vi "settings handler.vi"(7 "Operation":enum16{"Open", "Write", "Read", "Close"}(ring), 8 "error in (no error)":errorcluster, 9 "Paths write":cluster{"Android":path, "Version":path}, 11 "Write":T1={"COM"="", "baud rate"=115200, "data bits"=8, "parity"=enum."None", "stop bits"=10, "flow control"=enum."None", "delay"=50, "I/O channel"=""} {"stop bits" items=["1.0"=10, "1.5"=15, "2.0"=20]; "baud rate" max=921600; "data bits" max=16}) -> (0 "Error Out":errorcluster, 1 "Paths read":cluster{"Android":path, "Version":path}, 3 "Read":T1={"COM"="", "baud rate"=115200, "data bits"=8, "parity"=enum."None", "stop bits"=10, "flow control"=enum."None", "delay"=50, "I/O channel"=""} {"stop bits" items=["1.0"=10, "1.5"=15, "2.0"=20]; "baud rate" max=921600; "data bits" max=16})   [LabVIEW 2021]
uses:
  <vilib>/Utility/config.llb/Write Key (String).vi
  <vilib>/Utility/config.llb/Read Key (String).vi
  <vilib>/Utility/config.llb/Read Key (U32).vi
  <vilib>/Utility/config.llb/NI_LVConfig.lvlib
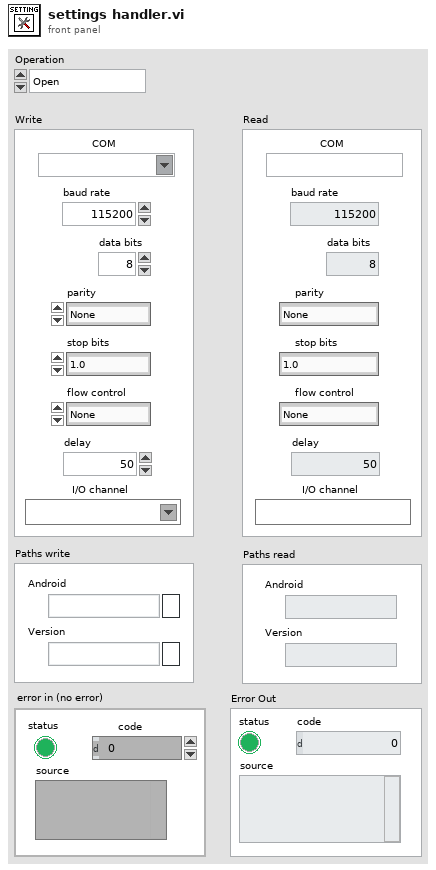
[diagram p1: front panel]
types:
  T1 = cluster{"COM":refnum<visa-resource-name>, "baud rate":u32, "data bits":u8, "parity":enum16{"None", "Odd", "Even", "Mark", "Space"}, "stop bits":u16, "flow control":enum16{"None", "XON/XOFF", "RTS/CTS", "DTR/DSR"}, "delay":u16, "I/O channel":refnum<k21>}
  T2 = typedef "NI_LVConfig.lvlib/Config Data RefNum.ctl" = refnum<k1>
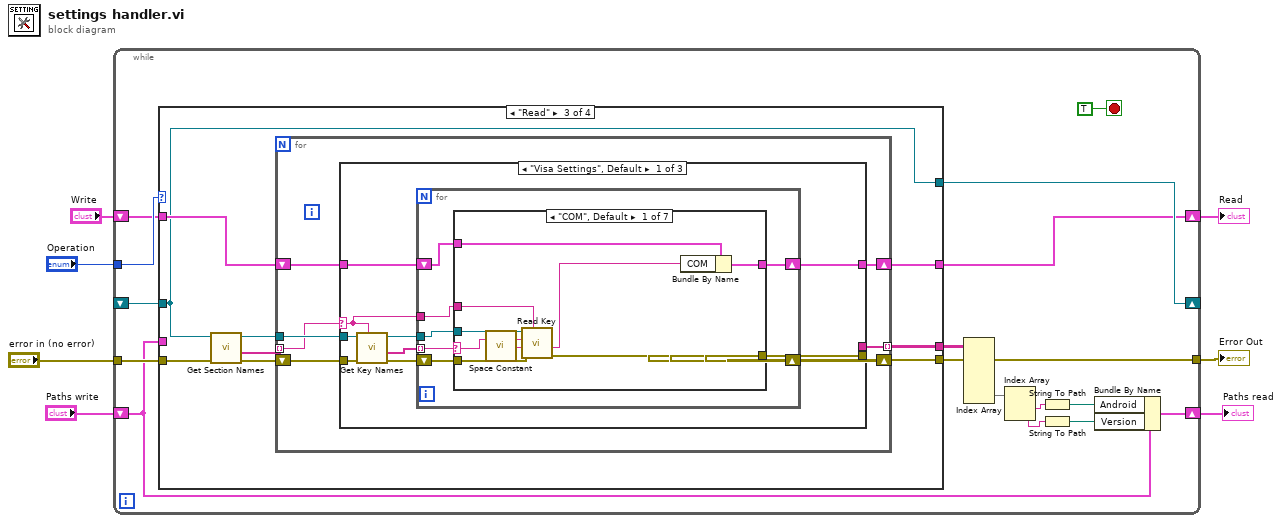
[diagram p0: block diagram]
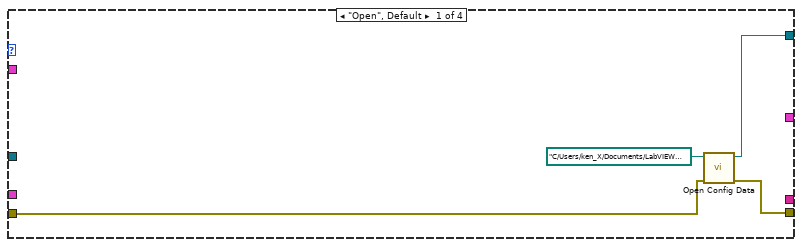
[diagram p2: hidden frame]
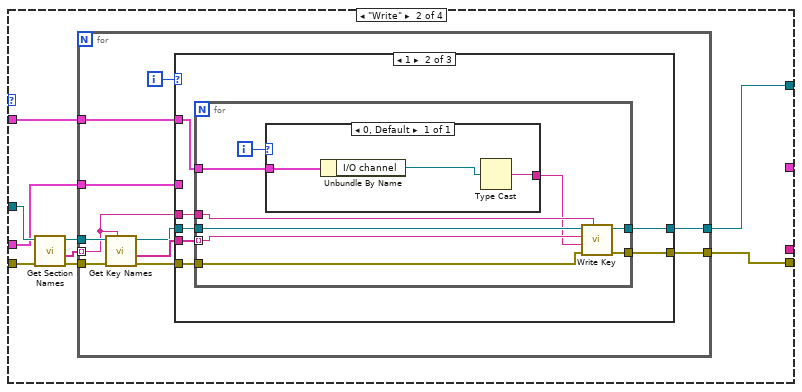
[diagram p3: hidden frame]
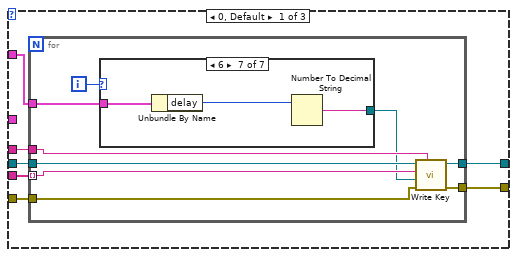
[diagram p4: hidden frame]
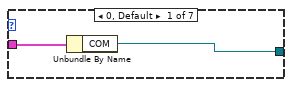
[diagram p5: hidden frame]
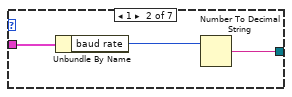
[diagram p6: hidden frame]
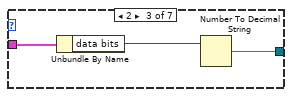
[diagram p7: hidden frame]
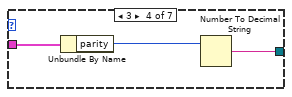
[diagram p8: hidden frame]
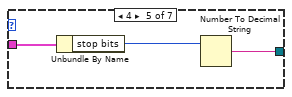
[diagram p9: hidden frame]
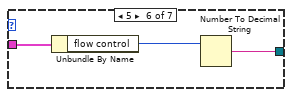
[diagram p10: hidden frame]
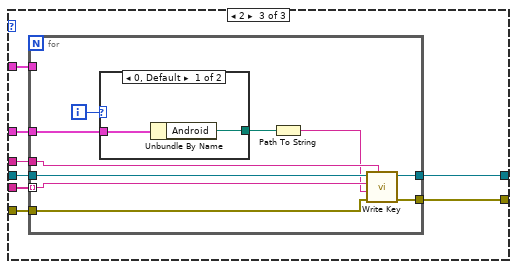
[diagram p11: hidden frame]
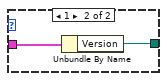
[diagram p12: hidden frame]
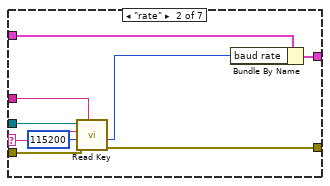
[diagram p13: hidden frame]
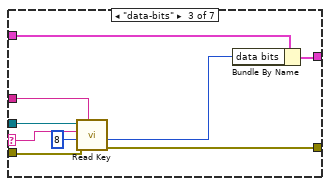
[diagram p14: hidden frame]
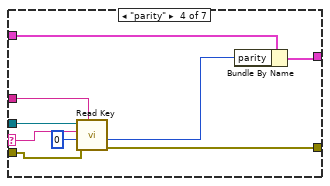
[diagram p15: hidden frame]
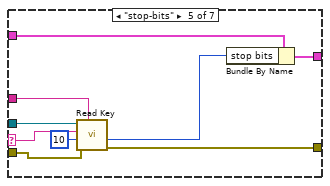
[diagram p16: hidden frame]
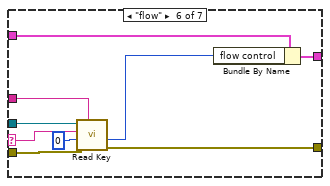
[diagram p17: hidden frame]
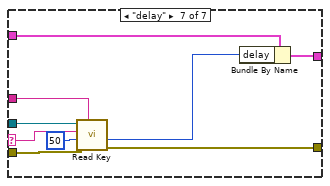
[diagram p18: hidden frame]
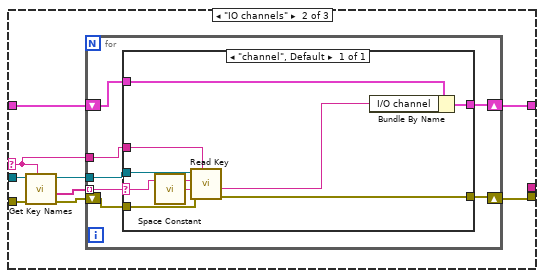
[diagram p19: hidden frame]
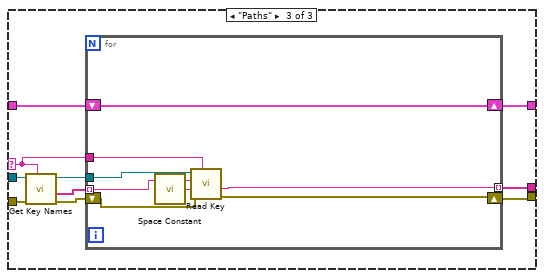
[diagram p20: hidden frame]
diagram:
  n1 = while {
    tunnel: "error in (no error)" -> [w23]
    tunnel: [w22] -> w6
    shift-right: [w21] -> _
    shift-left: _ -> [w19]
    shift-right: [w12] -> w3
    shift-left: "Write" -> [w17]
    tunnel: "Operation" -> [w18]
    shift-right: [w15] -> w1
    shift-left: "Paths write" -> [w16]
    stop <- TRUE stop-if-true
    n2 = case shown="\"Read\"" w18 {
      tunnel: w23 -> [w26 w33 w133 w265]
      tunnel: [w25 w29 w130 w264] -> w22
      tunnel: [w24 w30 w125 _] -> w21
      tunnel: w19 -> [_ w32 w125 w263]
      tunnel: w17 -> [_ w31 w128 _]
      tunnel: w16 -> [_ w28 _ _]
      tunnel: [_ _ w129 _] -> w12
      tunnel: [_ _ w127 _] -> w11
      frame "Open", Default {
        n3 = call <vilib>:"Open Config Data.vi"("error in (no error)"=w26, "configuration file path"=path "C:/Users/ken_X/Documents/LabVIEW projects/Project-A/settings/settings.ini" ("file path (use dialog)")) -> ("error out"=w25:errorcluster, "refnum"=w24:T2)  [unwired: 7 in, 1 out]
      }
      frame "Write" {
        n4 = call <vilib>:"Get Section Names.vi"("error in (no error)"=w33, "refnum"=w32) -> ("error out"=w34:errorcluster, "section names"=w36:string[], "refnum out"=w35:T2)  [unwired: 7 in]
        n5 = for {
          tunnel: w36 -> [w45] mode=indexing
          tunnel: w35 -> [w47]
          tunnel: w34 -> [w46]
          tunnel: [w41] -> w30
          tunnel: [w40] -> w29
          tunnel: w31 -> [w39]
          tunnel: w28 -> [w37]
          i -> [w38]
          n6 = call <vilib>:"Get Key Names.vi"("section"=w45, "error in (no error)"=w46, "refnum"=w47) -> ("error out"=w42:errorcluster, "key names"=w44:string[], "refnum out"=w43:T2)  [unwired: 5 in, 1 out]
          n7 = case shown="1" w38 {
            tunnel: w45 -> [w54 w90 w110]
            tunnel: w44 -> [w53 w89 w109]
            tunnel: w43 -> [w52 w88 w108]
            tunnel: w42 -> [w51 w87 w107]
            tunnel: [w50 w86 w106] -> w41
            tunnel: [w49 w85 w105] -> w40
            tunnel: w39 -> [w48 w84 w104]
            tunnel: w37 -> [_ _ w103]
            frame 0, Default {
              n8 = for {
                tunnel: w54 -> [w63]
                tunnel: w53 -> [w62] mode=indexing
                tunnel: w52 -> [w61]
                tunnel: w51 -> [w60]
                tunnel: [w59] -> w50
                tunnel: [w58] -> w49
                tunnel: w48 -> [w56]
                i -> [w57]
                n9 = case shown="6" w57 {
                  tunnel: w56 -> [w65 w68 w71 w74 w77 w80 w83]
                  tunnel: [w64 w66 w69 w72 w75 w78 w81] -> w55
                  frame 0, Default {
                    n10 = Unbundle By Name(w65) -> ("COM"=w64:refnum<visa-resource-name>)
                  }
                  frame 1 {
                    n11 = Unbundle By Name(w68) -> ("baud rate"=w67:u32)
                    n12 = Number To Decimal String(number=w67) -> (decimal integer string=w66:string)  [unwired: 1 in]
                  }
                  frame 2 {
                    n13 = Unbundle By Name(w71) -> ("data bits"=w70:u8)
                    n14 = Number To Decimal String(number=w70) -> (decimal integer string=w69:string)  [unwired: 1 in]
                  }
                  frame 3 {
                    n15 = Unbundle By Name(w74) -> ("parity"=w73:enum16{"None", "Odd", "Even", "Mark", "Space"})
                    n16 = Number To Decimal String(number=w73) -> (decimal integer string=w72:string)  [unwired: 1 in]
                  }
                  frame 4 {
                    n17 = Unbundle By Name(w77) -> ("stop bits"=w76:u16)
                    n18 = Number To Decimal String(number=w76) -> (decimal integer string=w75:string)  [unwired: 1 in]
                  }
                  frame 5 {
                    n19 = Unbundle By Name(w80) -> ("flow control"=w79:enum16{"None", "XON/XOFF", "RTS/CTS", "DTR/DSR"})
                    n20 = Number To Decimal String(number=w79) -> (decimal integer string=w78:string)  [unwired: 1 in]
                  }
                  frame 6 {
                    n21 = Unbundle By Name(w83) -> ("delay"=w82:u16)
                    n22 = Number To Decimal String(number=w82) -> (decimal integer string=w81:string)  [unwired: 1 in]
                  }
                }
                n23 = call-poly <vilib>:"Write Key.vi"("section"=w63, "error in (no error)"=w60, "value"=w55, "key"=w62, "refnum"=w61) -> ("error out"=w58:errorcluster, "refnum out"=w59:T2)  [unwired: 4 in, 1 out]
              }
            }
            frame 1 {
              n24 = for {
                tunnel: w90 -> [w99]
                tunnel: w89 -> [w98] mode=indexing
                tunnel: w88 -> [w97]
                tunnel: w87 -> [w96]
                tunnel: [w95] -> w86
                tunnel: [w94] -> w85
                tunnel: w84 -> [w92]
                i -> [w93]
                n25 = case shown="0, Default" w93 {
                  tunnel: w92 -> [w102]
                  tunnel: [w101] -> w91
                  frame 0, Default {
                    n26 = Unbundle By Name(w102) -> ("I/O channel"=w100:refnum<k21>)
                    n27 = Type Cast(x=w100) -> (*(type *) &x=w101:string)  [unwired: 1 in]
                  }
                }
                n28 = call-poly <vilib>:"Write Key.vi"("section"=w99, "error in (no error)"=w96, "value"=w91, "key"=w98, "refnum"=w97) -> ("error out"=w94:errorcluster, "refnum out"=w95:T2)  [unwired: 4 in, 1 out]
              }
            }
            frame 2 {
              n29 = for {
                tunnel: w110 -> [w120]
                tunnel: w109 -> [w119] mode=indexing
                tunnel: w108 -> [w118]
                tunnel: w107 -> [w117]
                tunnel: [w116] -> w106
                tunnel: [w115] -> w105
                tunnel: w104 -> [_]
                tunnel: w103 -> [w113]
                i -> [w114]
                n30 = case shown="0, Default" w114 {
                  tunnel: w113 -> [w121 w124]
                  tunnel: [w122 w123] -> w112
                  frame 0, Default {
                    n31 = Unbundle By Name(w121) -> ("Android"=w122:path)
                  }
                  frame 1 {
                    n32 = Unbundle By Name(w124) -> ("Version"=w123:path)
                  }
                }
                n33 = Path To String(path=w112) -> (string=w111:string)
                n34 = call-poly <vilib>:"Write Key.vi"("section"=w120, "error in (no error)"=w117, "value"=w111, "key"=w119, "refnum"=w118) -> ("error out"=w115:errorcluster, "refnum out"=w116:T2)  [unwired: 4 in, 1 out]
              }
            }
          }
        }
      }
      frame "Read" {
        n35 = call <vilib>:"Get Section Names.vi"("error in (no error)"=w133, "refnum"=w125) -> ("error out"=w131:errorcluster, "section names"=w132:string[], "refnum out"=w126:T2)  [unwired: 7 in]
        n36 = for {
          tunnel: w132 -> [w138] mode=indexing
          tunnel: w126 -> [w140]
          shift-right: [w137] -> w130
          shift-left: w131 -> [w139]
          shift-right: [w136] -> w129
          shift-left: w128 -> [w135]
          tunnel: [w134] -> w127 mode=indexing
          n37 = case shown="\"Visa Settings\", Default" w138 {
            selector: w138 -> [w144 w223 w249]
            tunnel: w140 -> [w149 w228 w254]
            tunnel: w139 -> [w148 w227 w253]
            tunnel: [w143 w222 w248] -> w137
            tunnel: [w142 w220 w246] -> w136
            tunnel: w135 -> [w141 w221 w247]
            tunnel: [_ _ w245] -> w134
            frame "Visa Settings", Default {
              n38 = call <vilib>:"Get Key Names.vi"("section"=w144, "error in (no error)"=w148, "refnum"=w149) -> ("error out"=w145:errorcluster, "key names"=w147:string[], "refnum out"=w146:T2)  [unwired: 5 in, 1 out]
              n39 = for {
                tunnel: w144 -> [w155]
                tunnel: w147 -> [w156] mode=indexing
                tunnel: w146 -> [w154]
                shift-right: [w152] -> w143
                shift-left: w145 -> [w153]
                shift-right: [w151] -> w142
                shift-left: w141 -> [w150]
                n40 = case shown="\"COM\", Default" w156 {
                  selector: w156 -> [w164 w173 w182 w191 w200 w209 w218]
                  tunnel: w155 -> [w165 w174 w183 w192 w201 w210 w219]
                  tunnel: w154 -> [w163 w172 w181 w184 w199 w208 w217]
                  tunnel: w153 -> [w162 w171 w180 w189 w197 w207 w216]
                  tunnel: [w160 w169 w178 w188 w196 w205 w214] -> w152
                  tunnel: w150 -> [w158 w168 w176 w186 w194 w203 w212]
                  tunnel: [w159 w167 w177 w187 w195 w204 w213] -> w151
                  frame "COM", Default {
                    n41 = call <vilib>:"Space Constant.vi"() -> ("String"=w161:string)
                    n42 = call-poly <vilib>:"Read Key.vi"("section"=w165, "error in (no error)"=w162, "default value"=w161, "key"=w164, "refnum"=w163) -> ("error out"=w160:errorcluster, "value"=w157:string)  [unwired: 3 in, 2 out]
                    n43 = Bundle By Name(cluster=w158, "COM"=w157) -> (w159:T1)
                  }
                  frame "rate" {
                    n44 = call-poly <vilib>:"Read Key.vi"("section"=w174, "error in (no error)"=w171, "default value"=u32 115200, "key"=w173, "refnum"=w172) -> ("error out"=w169:errorcluster, "value"=w166:u32)  [unwired: 3 in, 2 out]
                    n45 = Bundle By Name(cluster=w168, "baud rate"=w166) -> (w167:T1)
                  }
                  frame "data-bits" {
                    n46 = call-poly <vilib>:"Read Key.vi"("section"=w183, "error in (no error)"=w180, "default value"=u32 8, "key"=w182, "refnum"=w181) -> ("error out"=w178:errorcluster, "value"=w175:u32)  [unwired: 3 in, 2 out]
                    n47 = Bundle By Name(cluster=w176, "data bits"=w175) -> (w177:T1)
                  }
                  frame "parity" {
                    n48 = call-poly <vilib>:"Read Key.vi"("section"=w192, "error in (no error)"=w189, "default value"=u32 0, "key"=w191, "refnum"=w184) -> ("error out"=w188:errorcluster, "value"=w185:u32)  [unwired: 3 in, 2 out]
                    n49 = Bundle By Name(cluster=w186, "parity"=w185) -> (w187:T1)
                  }
                  frame "stop-bits" {
                    n50 = call-poly <vilib>:"Read Key.vi"("section"=w201, "error in (no error)"=w197, "default value"=u32 10, "key"=w200, "refnum"=w199) -> ("error out"=w196:errorcluster, "value"=w193:u32)  [unwired: 3 in, 2 out]
                    n51 = Bundle By Name(cluster=w194, "stop bits"=w193) -> (w195:T1)
                  }
                  frame "flow" {
                    n52 = call-poly <vilib>:"Read Key.vi"("section"=w210, "error in (no error)"=w207, "default value"=u32 0, "key"=w209, "refnum"=w208) -> ("error out"=w205:errorcluster, "value"=w202:u32)  [unwired: 3 in, 2 out]
                    n53 = Bundle By Name(cluster=w203, "flow control"=w202) -> (w204:T1)
                  }
                  frame "delay" {
                    n54 = call-poly <vilib>:"Read Key.vi"("section"=w219, "error in (no error)"=w216, "default value"=u32 50, "key"=w218, "refnum"=w217) -> ("error out"=w214:errorcluster, "value"=w211:u32)  [unwired: 3 in, 2 out]
                    n55 = Bundle By Name(cluster=w212, "delay"=w211) -> (w213:T1)
                  }
                }
              }
            }
            frame "IO channels" {
              n56 = call <vilib>:"Get Key Names.vi"("section"=w223, "error in (no error)"=w227, "refnum"=w228) -> ("error out"=w224:errorcluster, "key names"=w226:string[], "refnum out"=w225:T2)  [unwired: 5 in, 1 out]
              n57 = for {
                tunnel: w223 -> [w234]
                tunnel: w226 -> [w235] mode=indexing
                tunnel: w225 -> [w233]
                shift-right: [w231] -> w222
                shift-left: w224 -> [w232]
                shift-right: [w229] -> w220
                shift-left: w221 -> [w230]
                n58 = case shown="\"channel\", Default" w235 {
                  selector: w235 -> [w243]
                  tunnel: w234 -> [w244]
                  tunnel: w233 -> [w242]
                  tunnel: w232 -> [w240]
                  tunnel: [w239] -> w231
                  tunnel: [w238] -> w229
                  tunnel: w230 -> [w237]
                  frame "channel", Default {
                    n59 = call <vilib>:"Space Constant.vi"() -> ("String"=w241:string)
                    n60 = call-poly <vilib>:"Read Key.vi"("section"=w244, "error in (no error)"=w240, "default value"=w241, "key"=w243, "refnum"=w242) -> ("error out"=w239:errorcluster, "value"=w236:string)  [unwired: 3 in, 2 out]
                    n61 = Bundle By Name(cluster=w237, "I/O channel"=w236) -> (w238:T1)
                  }
                }
              }
            }
            frame "Paths" {
              n62 = call <vilib>:"Get Key Names.vi"("section"=w249, "error in (no error)"=w253, "refnum"=w254) -> ("error out"=w250:errorcluster, "key names"=w252:string[], "refnum out"=w251:T2)  [unwired: 5 in, 1 out]
              n63 = for {
                tunnel: w249 -> [w261]
                tunnel: w252 -> [w262] mode=indexing
                tunnel: w251 -> [w260]
                shift-right: [w258] -> w248
                shift-left: w250 -> [w259]
                shift-right: [w256] -> w246
                shift-left: w247 -> [w256]
                tunnel: [w255] -> w245 mode=indexing
                n64 = call <vilib>:"Space Constant.vi"() -> ("String"=w257:string)
                n65 = call-poly <vilib>:"Read Key.vi"("section"=w261, "error in (no error)"=w259, "default value"=w257, "key"=w262, "refnum"=w260) -> ("error out"=w258:errorcluster, "value"=w255:string)  [unwired: 3 in, 2 out]
              }
            }
          }
        }
      }
      frame "Close" {
        n66 = call <vilib>:"Close Config Data.vi"("error in (no error)"=w265, "refnum"=w263) -> ("error out"=w264:errorcluster)  [unwired: 8 in, 1 out]
      }
    }
    n67 = Index Array(array=w11) -> (element #3=w10:string[])  [unwired: 6 in, 2 out]
    n68 = Index Array(array=w10) -> (element #1=w8:string, element #2=w9:string)  [unwired: 2 in]
    n69 = String To Path(string=w8) -> (path=w14:path)
    n70 = String To Path(string=w9) -> (path=w13:path)
    n71 = Bundle By Name(cluster=w16, "Android"=w14, "Version"=w13) -> (w15:cluster{"Android":path, "Version":path})
  }
  "Error Out" <- w6
  "Read" <- w3
  "Paths read" <- w1
